vi "Is Auto Populating Folder.vi"(0 "Refnum in":refnum<k20>) -> (4 "Auto Populating Folder?":bool)   [LabVIEW 2016]
uses:
  <vilib>/xml/Close Reference(Node).vi
  <vilib>/xml/Close Reference(NNMap).vi
  <resource>/objmgr/DOMUserDefRef.rc
  <vilib>/xml/NI_XML.lvlib
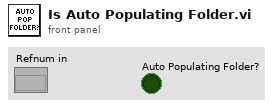
[diagram p1: front panel]
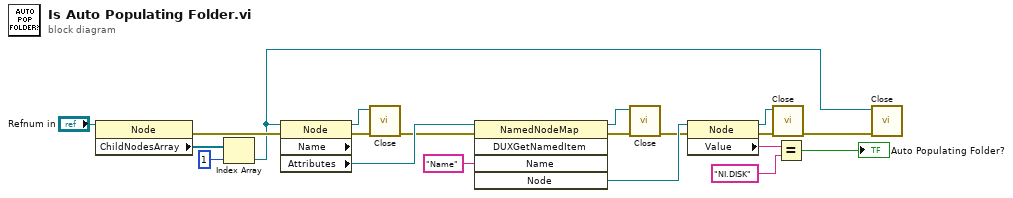
[diagram p0: block diagram]
diagram:
  n1 = property class="Node"(reference="Refnum in") -> (error out=w19:errorcluster, "ChildNodesArray"=w2:refnum<k20>[])  [unwired: 1 in, 1 out]
  n2 = Index Array(array=w2, index=1) -> (element=w1:refnum<k20>)
  n3 = property class="Node" props=["Name", "Attributes"](reference=w1, error in=w19) -> (reference out=w12:refnum<k20>, error out=w14:errorcluster, "Attributes"=w16:refnum<k20>)  [unwired: 1 out]
  n4 = call-poly <vilib>:"Close.vi"("error in (no error)"=w14, "node"=w12) -> ("error out"=w13:errorcluster)  [unwired: 7 in]
  n5 = invoke class="NamedNodeMap" method="DUXGetNamedItem"(reference=w16, error in=w13, "Name"="Name") -> (reference out=w10:refnum<k20>, error out=w9:errorcluster, "Node"=w11:refnum<k20>)  [unwired: 2 in, 2 out]
  n6 = call-poly <vilib>:"Close.vi"("error in (no error)"=w9, "named node map"=w10) -> ("error out"=w8:errorcluster)  [unwired: 7 in]
  n7 = property class="Node"(reference=w11, error in=w8) -> (reference out=w4:refnum<k20>, error out=w5:errorcluster, "Value"=w7:string)
  n8 = call-poly <vilib>:"Close.vi"("error in (no error)"=w5, "node"=w4) -> ("error out"=w17:errorcluster)  [unwired: 7 in]
  n9 = Equal?(x=w7, y="NI.DISK") -> (x = y?=→"Auto Populating Folder?":bool)
  n10 = call-poly <vilib>:"Close.vi"("error in (no error)"=w17, "node"=w1) -> ()  [unwired: 7 in, 1 out]
